vi "getTATUpdateData.vi"(9 "time":i32, 10 "Status":string, 11 "step":string) -> (2 "updateData":string)   [LabVIEW 2012]
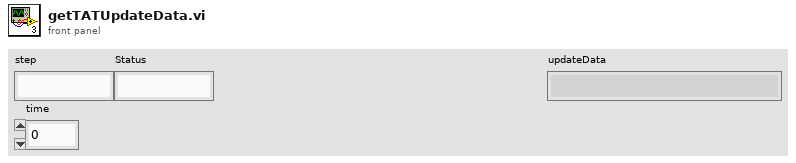
[diagram p1: front panel]
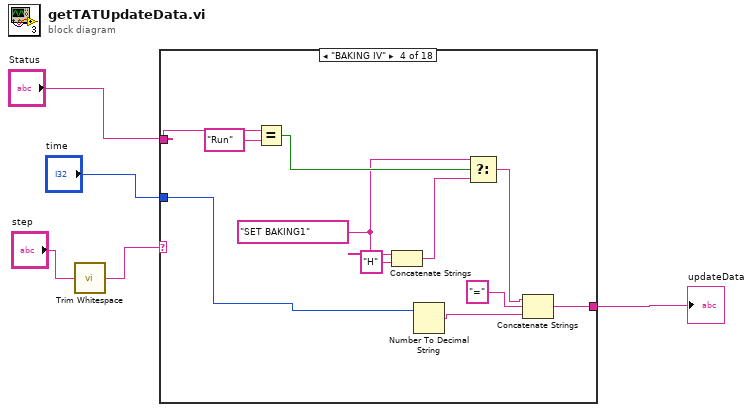
[diagram p0: block diagram]
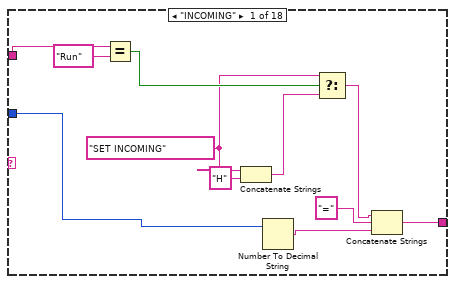
[diagram p2: hidden frame]
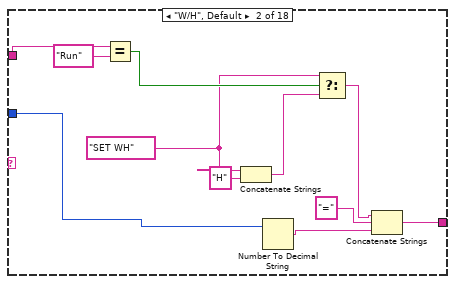
[diagram p3: hidden frame]
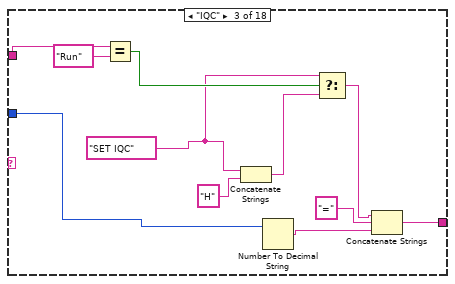
[diagram p4: hidden frame]
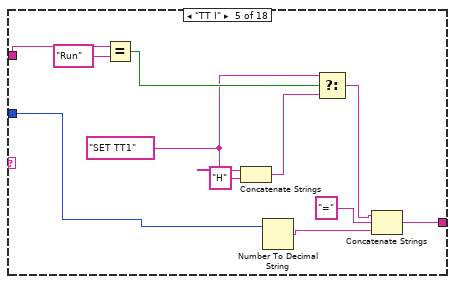
[diagram p5: hidden frame]
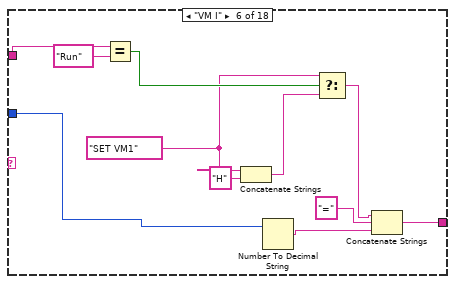
[diagram p6: hidden frame]
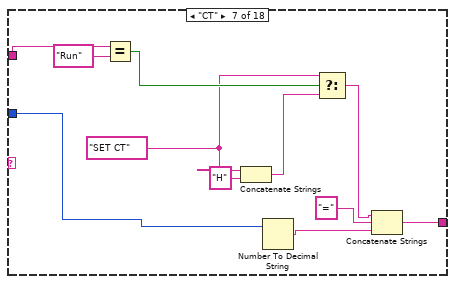
[diagram p7: hidden frame]
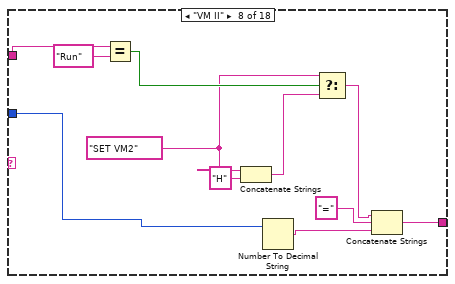
[diagram p8: hidden frame]
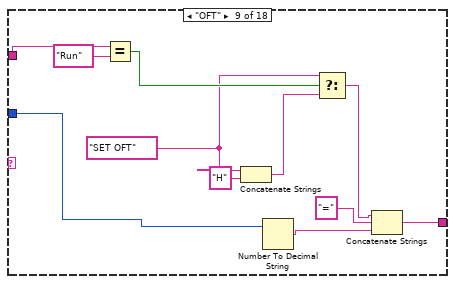
[diagram p9: hidden frame]
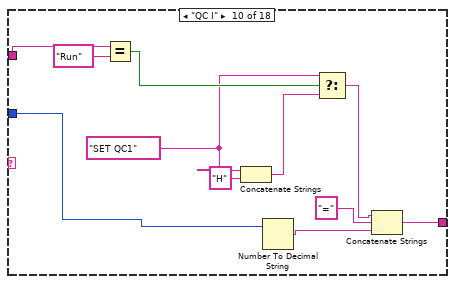
[diagram p10: hidden frame]
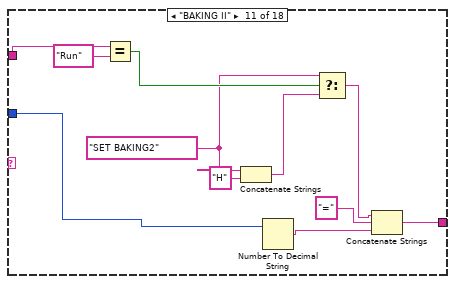
[diagram p11: hidden frame]
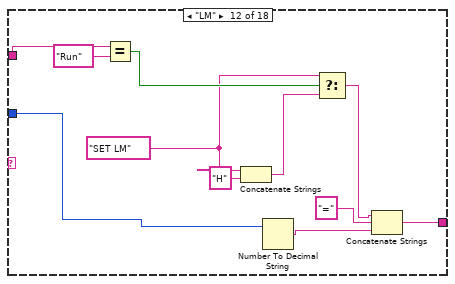
[diagram p12: hidden frame]
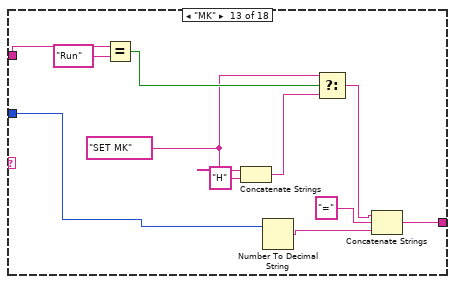
[diagram p13: hidden frame]
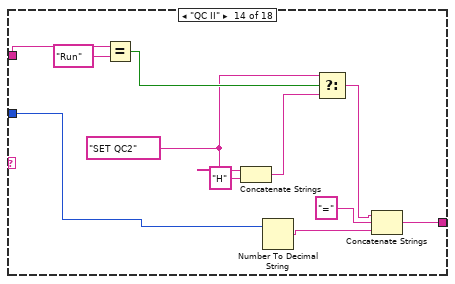
[diagram p14: hidden frame]
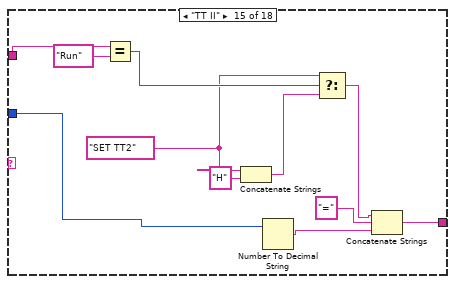
[diagram p15: hidden frame]
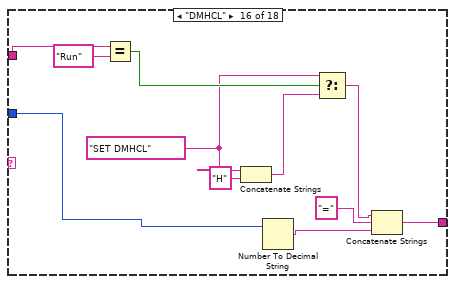
[diagram p16: hidden frame]
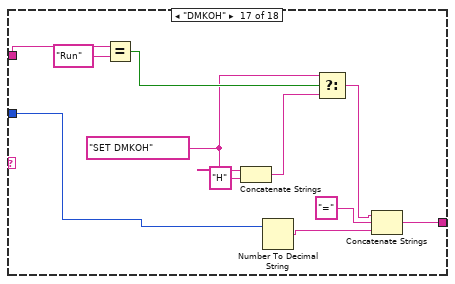
[diagram p17: hidden frame]
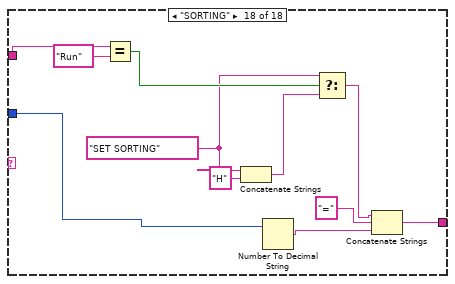
[diagram p18: hidden frame]
diagram:
  n1 = call <vilib>:"Trim Whitespace.vi"("string"="step") -> ("trimmed string"=w1:string)  [unwired: 1 in]
  n2 = case shown="\"BAKING IV\"" w1 {
    tunnel: "time" -> [w9 w20 w31 w42 w53 w64 w75 w86 w97 w108 w119 w130 w141 w152 w163 w174 w185 w196]
    tunnel: "Status" -> [w16 w27 w38 w49 w60 w71 w82 w93 w104 w115 w126 w137 w148 w159 w170 w181 w192 w203]
    tunnel: [w6 w17 w28 w39 w50 w61 w72 w83 w94 w105 w116 w127 w138 w149 w160 w171 w182 w193] -> w3
    frame "INCOMING" {
      w12 = "SET INCOMING"
      n3 = Equal?(x=w16, y="Run") -> (x = y?=w13:bool)
      n4 = Concatenate Strings(w12, "H" ("string")) -> (w11:string)
      n5 = Number To Decimal String(number=w9) -> (decimal integer string=w7:string)  [unwired: 1 in]
      n6 = Select(t=w12, s=w13, f=w11) -> (s? t:f=w10:string)
      n7 = Concatenate Strings(w10, "=" ("string"), w7) -> (w6:string)
    }
    frame "W/H", Default {
      w23 = "SET WH"
      n8 = Equal?(x=w27, y="Run") -> (x = y?=w24:bool)
      n9 = Concatenate Strings(w23, "H" ("string")) -> (w22:string)
      n10 = Number To Decimal String(number=w20) -> (decimal integer string=w18:string)  [unwired: 1 in]
      n11 = Select(t=w23, s=w24, f=w22) -> (s? t:f=w21:string)
      n12 = Concatenate Strings(w21, "=" ("string"), w18) -> (w17:string)
    }
    frame "IQC" {
      w34 = "SET IQC"
      n13 = Equal?(x=w38, y="Run") -> (x = y?=w35:bool)
      n14 = Concatenate Strings(w34, "H" ("string")) -> (w33:string)
      n15 = Number To Decimal String(number=w31) -> (decimal integer string=w29:string)  [unwired: 1 in]
      n16 = Select(t=w34, s=w35, f=w33) -> (s? t:f=w32:string)
      n17 = Concatenate Strings(w32, "=" ("string"), w29) -> (w28:string)
    }
    frame "BAKING IV" {
      w45 = "SET BAKING1"
      n18 = Equal?(x=w49, y="Run") -> (x = y?=w46:bool)
      n19 = Concatenate Strings(w45, "H" ("string")) -> (w44:string)
      n20 = Number To Decimal String(number=w42) -> (decimal integer string=w40:string)  [unwired: 1 in]
      n21 = Select(t=w45, s=w46, f=w44) -> (s? t:f=w43:string)
      n22 = Concatenate Strings(w43, "=" ("string"), w40) -> (w39:string)
    }
    frame "TT I" {
      w56 = "SET TT1"
      n23 = Equal?(x=w60, y="Run") -> (x = y?=w57:bool)
      n24 = Concatenate Strings(w56, "H" ("string")) -> (w55:string)
      n25 = Number To Decimal String(number=w53) -> (decimal integer string=w51:string)  [unwired: 1 in]
      n26 = Select(t=w56, s=w57, f=w55) -> (s? t:f=w54:string)
      n27 = Concatenate Strings(w54, "=" ("string"), w51) -> (w50:string)
    }
    frame "VM I" {
      w67 = "SET VM1"
      n28 = Equal?(x=w71, y="Run") -> (x = y?=w68:bool)
      n29 = Concatenate Strings(w67, "H" ("string")) -> (w66:string)
      n30 = Number To Decimal String(number=w64) -> (decimal integer string=w62:string)  [unwired: 1 in]
      n31 = Select(t=w67, s=w68, f=w66) -> (s? t:f=w65:string)
      n32 = Concatenate Strings(w65, "=" ("string"), w62) -> (w61:string)
    }
    frame "CT" {
      w78 = "SET CT"
      n33 = Equal?(x=w82, y="Run") -> (x = y?=w79:bool)
      n34 = Concatenate Strings(w78, "H" ("string")) -> (w77:string)
      n35 = Number To Decimal String(number=w75) -> (decimal integer string=w73:string)  [unwired: 1 in]
      n36 = Select(t=w78, s=w79, f=w77) -> (s? t:f=w76:string)
      n37 = Concatenate Strings(w76, "=" ("string"), w73) -> (w72:string)
    }
    frame "VM II" {
      w89 = "SET VM2"
      n38 = Equal?(x=w93, y="Run") -> (x = y?=w90:bool)
      n39 = Concatenate Strings(w89, "H" ("string")) -> (w88:string)
      n40 = Number To Decimal String(number=w86) -> (decimal integer string=w84:string)  [unwired: 1 in]
      n41 = Select(t=w89, s=w90, f=w88) -> (s? t:f=w87:string)
      n42 = Concatenate Strings(w87, "=" ("string"), w84) -> (w83:string)
    }
    frame "OFT" {
      w100 = "SET OFT"
      n43 = Equal?(x=w104, y="Run") -> (x = y?=w101:bool)
      n44 = Concatenate Strings(w100, "H" ("string")) -> (w99:string)
      n45 = Number To Decimal String(number=w97) -> (decimal integer string=w95:string)  [unwired: 1 in]
      n46 = Select(t=w100, s=w101, f=w99) -> (s? t:f=w98:string)
      n47 = Concatenate Strings(w98, "=" ("string"), w95) -> (w94:string)
    }
    frame "QC I" {
      w111 = "SET QC1"
      n48 = Equal?(x=w115, y="Run") -> (x = y?=w112:bool)
      n49 = Concatenate Strings(w111, "H" ("string")) -> (w110:string)
      n50 = Number To Decimal String(number=w108) -> (decimal integer string=w106:string)  [unwired: 1 in]
      n51 = Select(t=w111, s=w112, f=w110) -> (s? t:f=w109:string)
      n52 = Concatenate Strings(w109, "=" ("string"), w106) -> (w105:string)
    }
    frame "BAKING II" {
      w122 = "SET BAKING2"
      n53 = Equal?(x=w126, y="Run") -> (x = y?=w123:bool)
      n54 = Concatenate Strings(w122, "H" ("string")) -> (w121:string)
      n55 = Number To Decimal String(number=w119) -> (decimal integer string=w117:string)  [unwired: 1 in]
      n56 = Select(t=w122, s=w123, f=w121) -> (s? t:f=w120:string)
      n57 = Concatenate Strings(w120, "=" ("string"), w117) -> (w116:string)
    }
    frame "LM" {
      w133 = "SET LM"
      n58 = Equal?(x=w137, y="Run") -> (x = y?=w134:bool)
      n59 = Concatenate Strings(w133, "H" ("string")) -> (w132:string)
      n60 = Number To Decimal String(number=w130) -> (decimal integer string=w128:string)  [unwired: 1 in]
      n61 = Select(t=w133, s=w134, f=w132) -> (s? t:f=w131:string)
      n62 = Concatenate Strings(w131, "=" ("string"), w128) -> (w127:string)
    }
    frame "MK" {
      w144 = "SET MK"
      n63 = Equal?(x=w148, y="Run") -> (x = y?=w145:bool)
      n64 = Concatenate Strings(w144, "H" ("string")) -> (w143:string)
      n65 = Number To Decimal String(number=w141) -> (decimal integer string=w139:string)  [unwired: 1 in]
      n66 = Select(t=w144, s=w145, f=w143) -> (s? t:f=w142:string)
      n67 = Concatenate Strings(w142, "=" ("string"), w139) -> (w138:string)
    }
    frame "QC II" {
      w155 = "SET QC2"
      n68 = Equal?(x=w159, y="Run") -> (x = y?=w156:bool)
      n69 = Concatenate Strings(w155, "H" ("string")) -> (w154:string)
      n70 = Number To Decimal String(number=w152) -> (decimal integer string=w150:string)  [unwired: 1 in]
      n71 = Select(t=w155, s=w156, f=w154) -> (s? t:f=w153:string)
      n72 = Concatenate Strings(w153, "=" ("string"), w150) -> (w149:string)
    }
    frame "TT II" {
      w166 = "SET TT2"
      n73 = Equal?(x=w170, y="Run") -> (x = y?=w167:bool)
      n74 = Concatenate Strings(w166, "H" ("string")) -> (w165:string)
      n75 = Number To Decimal String(number=w163) -> (decimal integer string=w161:string)  [unwired: 1 in]
      n76 = Select(t=w166, s=w167, f=w165) -> (s? t:f=w164:string)
      n77 = Concatenate Strings(w164, "=" ("string"), w161) -> (w160:string)
    }
    frame "DMHCL" {
      w177 = "SET DMHCL"
      n78 = Equal?(x=w181, y="Run") -> (x = y?=w178:bool)
      n79 = Concatenate Strings(w177, "H" ("string")) -> (w176:string)
      n80 = Number To Decimal String(number=w174) -> (decimal integer string=w172:string)  [unwired: 1 in]
      n81 = Select(t=w177, s=w178, f=w176) -> (s? t:f=w175:string)
      n82 = Concatenate Strings(w175, "=" ("string"), w172) -> (w171:string)
    }
    frame "DMKOH" {
      w188 = "SET DMKOH"
      n83 = Equal?(x=w192, y="Run") -> (x = y?=w189:bool)
      n84 = Concatenate Strings(w188, "H" ("string")) -> (w187:string)
      n85 = Number To Decimal String(number=w185) -> (decimal integer string=w183:string)  [unwired: 1 in]
      n86 = Select(t=w188, s=w189, f=w187) -> (s? t:f=w186:string)
      n87 = Concatenate Strings(w186, "=" ("string"), w183) -> (w182:string)
    }
    frame "SORTING" {
      w199 = "SET SORTING"
      n88 = Equal?(x=w203, y="Run") -> (x = y?=w200:bool)
      n89 = Concatenate Strings(w199, "H" ("string")) -> (w198:string)
      n90 = Number To Decimal String(number=w196) -> (decimal integer string=w194:string)  [unwired: 1 in]
      n91 = Select(t=w199, s=w200, f=w198) -> (s? t:f=w197:string)
      n92 = Concatenate Strings(w197, "=" ("string"), w194) -> (w193:string)
    }
  }
  "updateData" <- w3
